vi "Create.vi"(7 "Sender":refnum<class "Sender.lvclass">, 9 "jettl":refnum<class "jettl.lvclass">, 10 "Self Alias":string, 11 "Create in":refnum<class "Create.lvclass">) -> (3 "Create out":refnum<class "Create.lvclass">)   [LabVIEW 2021, in "Create Msg Strategy.lvlib" / "Create.lvclass"]
uses:
  Create.lvclass
  jettl/jettl/jettl.lvclass
  jettl/Sender/Sender/Sender.lvclass
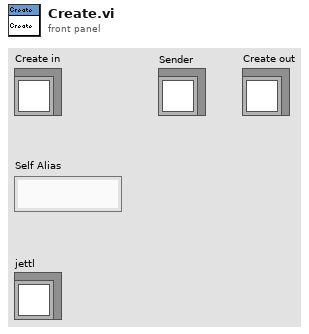
[diagram p1: front panel]
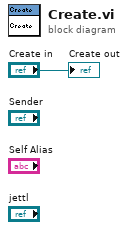
[diagram p0: block diagram]
diagram:
  "Create out" <- "Create in"
